vi "Launch Nested Actors.vi"(8 "error in (no error)":errorcluster, 11 "MusicManagerActor in":refnum<class "MusicManagerActor.lvclass">) -> (0 "error out":errorcluster, 3 "MusicManagerActor out":refnum<class "MusicManagerActor.lvclass">, 5 "Nested Actor Enqueuers":T1)   [LabVIEW 2015, in "MusicManagerActor.lvlib" / "MusicManagerActor.lvclass"]
uses:
  MusicManagerActor.lvclass
  Nested Actors Enqueuers.ctl
  <vilib>/ActorFramework/Message Enqueuer/Message Enqueuer.lvclass
  SongBrowserActor/SongBrowserActor/SongBrowserActor.lvclass
  SongQueueActor/SongQueueActor/SongQueueActor.lvclass
  AlbumImageActor/AlbumImageActor/AlbumImageActor.lvclass
  <vilib>/ActorFramework/Actor/Actor.lvclass/Actor.ctl
  <vilib>/ActorFramework/Message Enqueuer/Message Enqueuer.lvclass/Message Enqueuer.ctl
  MusicManagerActor.lvclass/MusicManagerActor.ctl
  SongQueueActor/SongQueueActor/SongQueueActor.lvclass/SongQueueActor.ctl
  <vilib>/ActorFramework/Message Enqueuer/Init from Existing Queue.vi
  <vilib>/ActorFramework/Actor/Actor.lvclass
  SongBrowserActor/SongBrowserActor Messages/Embed Actor Core In Subpanel Msg/Embed Actor Core In Subpanel Msg.lvclass
  SongQueueActor/SongQueueActor Messages/Embed Actor Core In Subpanel Msg/Embed Actor Core In Subpanel Msg.lvclass
  AlbumImageActor/AlbumImageActor Messages/Embed Actor Core In Subpanel Msg/Embed Actor Core In Subpanel Msg.lvclass
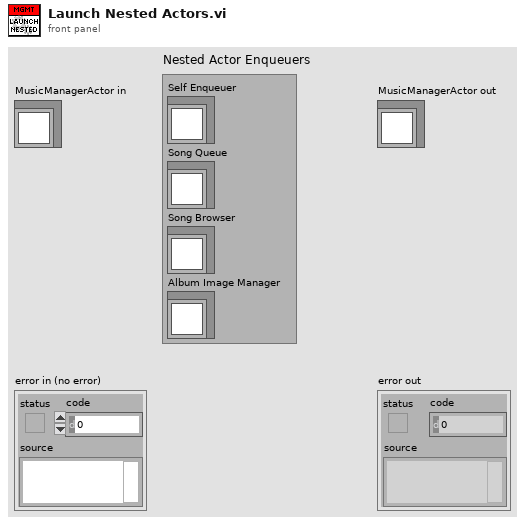
[diagram p1: front panel]
types:
  T1 = typedef "MusicManagerActor.lvlib/MusicManagerActor.lvclass/Nested Actors Enqueuers.ctl" = cluster{"Self Enqueuer":refnum<class "Message Enqueuer.lvclass">, "Song Queue":refnum<class "Message Enqueuer.lvclass">, "Song Browser":refnum<class "Message Enqueuer.lvclass">, "Album Image Manager":refnum<class "Message Enqueuer.lvclass">}
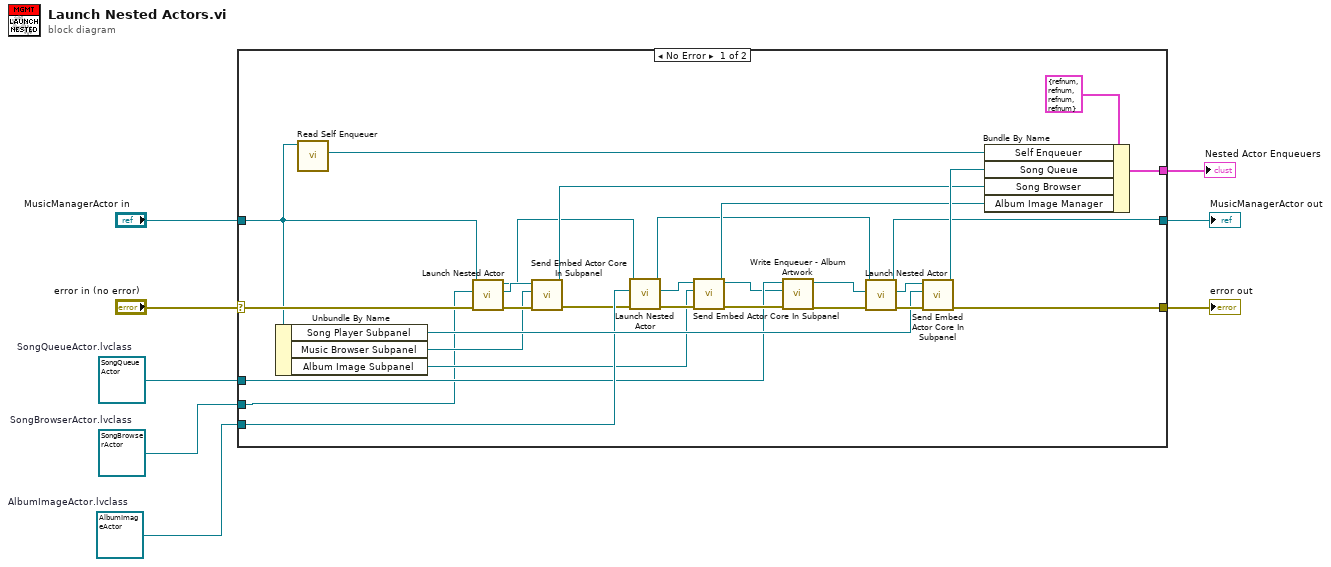
[diagram p0: block diagram]
diagram:
  w1 = refnum<class "AlbumImageActor.lvclass"> refnum  # AlbumImageActor.lvclass
  w2 = refnum<class "SongQueueActor.lvclass"> refnum  # SongQueueActor.lvclass
  w3 = refnum<class "SongBrowserActor.lvclass"> refnum  # SongBrowserActor.lvclass
  n1 = case shown="No Error" "error in (no error)" {
    selector: "error in (no error)" -> [w21 w38]
    tunnel: [w10 w38] -> w7
    tunnel: [w11 w37] -> w5
    tunnel: "MusicManagerActor in" -> [w20 w37]
    tunnel: [w35 _] -> w4
    tunnel: w2 -> [w16 _]
    tunnel: w3 -> [w9 _]
    tunnel: w1 -> [w25 _]
    frame No Error {
      n2 = Unbundle By Name(w20) -> ("Song Player Subpanel"=w28:refnum<vi>, "Music Browser Subpanel"=w27:refnum<vi>, "Album Image Subpanel"=w22:refnum<vi>)
      n3 = call <vilib>:"Read Self Enqueuer.vi"("Actor"=w20) -> ("Self Enqueuer"=w26:refnum<class "Message Enqueuer.lvclass">)  [unwired: 10 in]
      n4 = call <vilib>:"Launch Nested Actor.vi"("error in (no error)"=w21, "Nested Actor"=w9, "Caller Actor in"=w20) -> ("error out"=w34:errorcluster, "Nested Actor's Enqueuer"=w33:refnum<class "Message Enqueuer.lvclass">, "Caller Actor out"=w19:refnum<class "MusicManagerActor.lvclass">)  [unwired: 6 in]
      n5 = call "Send Embed Actor Core In Subpanel.vi"("error in (no error)"=w34, "Subpanel"=w27, "Message Enqueuer in"=w33) -> ("error out"=w18:errorcluster, "Message Enqueuer out"=w29:refnum<class "Message Enqueuer.lvclass">)  [unwired: 7 in]
      n6 = call <vilib>:"Launch Nested Actor.vi"("error in (no error)"=w18, "Nested Actor"=w25, "Caller Actor in"=w19) -> ("error out"=w24:errorcluster, "Nested Actor's Enqueuer"=w23:refnum<class "Message Enqueuer.lvclass">, "Caller Actor out"=w12:refnum<class "MusicManagerActor.lvclass">)  [unwired: 6 in]
      n7 = call "Send Embed Actor Core In Subpanel.vi"("error in (no error)"=w24, "Subpanel"=w22, "Message Enqueuer in"=w23) -> ("error out"=w17:errorcluster, "Message Enqueuer out"=w14:refnum<class "Message Enqueuer.lvclass">)  [unwired: 7 in]
      n8 = call "Write Enqueuer - Album Artwork.vi"("error in (no error)"=w17, "Actor Framework:Message Enqueuer"=w14, "SongQueueActor in"=w16) -> ("error out"=w13:errorcluster, "SongQueueActor out"=w15:refnum<class "SongQueueActor.lvclass">)  [unwired: 7 in]
      n9 = call <vilib>:"Launch Nested Actor.vi"("error in (no error)"=w13, "Nested Actor"=w15, "Caller Actor in"=w12) -> ("error out"=w32:errorcluster, "Nested Actor's Enqueuer"=w31:refnum<class "Message Enqueuer.lvclass">, "Caller Actor out"=w11:refnum<class "MusicManagerActor.lvclass">)  [unwired: 6 in]
      n10 = call "Send Embed Actor Core In Subpanel.vi"("error in (no error)"=w32, "Subpanel"=w28, "Message Enqueuer in"=w31) -> ("error out"=w10:errorcluster, "Message Enqueuer out"=w30:refnum<class "Message Enqueuer.lvclass">)  [unwired: 7 in]
      n11 = Bundle By Name(cluster=T1 {"Self Enqueuer"=refnum, "Song Queue"=refnum, "Song Browser"=refnum, "Album Image Manager"=refnum} ("Nested Actor Enqueuers"), "Self Enqueuer"=w26, "Song Queue"=w30, "Song Browser"=w29, "Album Image Manager"=w14) -> (w35:T1)
    }
    frame Error {
    }
  }
  "error out" <- w7
  "MusicManagerActor out" <- w5
  "Nested Actor Enqueuers" <- w4
